vi "String to Complex.vi"(11 "string":string) -> (3 "complex number":cdb)   [LabVIEW 2020, in "GOLPI library.lvlib"]
doc: "Converts string with complex number into complex double format. VI suppose complex parts are in %e format and are separated by ' + ' or ' - ' (with spaces). In the case of parse error output is NaN +NaN i."
uses:
  GOLPI library.lvlib
  <vilib>/regexp/Match Regular Expression.xnode
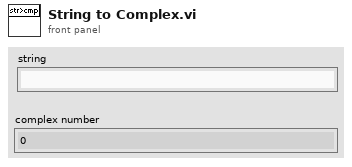
[diagram p1: front panel]
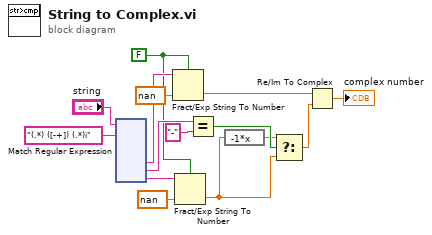
[diagram p0: block diagram]
diagram:
  w7 = FALSE ("use system decimal point (T)")
  n1 = xnode "Match Regular Expression"("input string"="string", "regular expression"="(.*) ([-+]) (.*)i") -> ("submatch 1"=w10:string, "submatch 2"=w12:string, "submatch 3"=w11:string)  [unwired: 4 in, 5 out]
  n2 = Fract/Exp String To Number(use system decimal point (T)=w7, string=w10, default (0 dbl)=nan ("default (0 DBL)")) -> (number=w5:dbl)  [unwired: 1 in, 1 out]
  n3 = Fract/Exp String To Number(use system decimal point (T)=w7, string=w11, default (0 dbl)=nan ("default (0 DBL)")) -> (number=w4:dbl)  [unwired: 1 in, 1 out]
  n4 = Equal?(x=w12, y="-") -> (x = y?=w14:bool)
  n5 = expression code="-1*x"(w4) -> (w3:dbl)
  n6 = Select(t=w3, s=w14, f=w4) -> (s? t:f=w15:dbl)
  n7 = Re/Im To Complex(1:w15, 2:w5) -> (0:→"complex number":cdb)
